vi "ResetBoard.vi"() -> ()   [LabVIEW 2020]
uses:
  _controls/hwEntry_actions.ctl
  AIM664LV.lvlib
panel:
  in  "board":u32
  out "error out":errorcluster
  out "Board Control Out":T1 {"SharedMemFree" format="%x"; "GlobalMemFree" format="%x"; "ExpertMode" items=["FDX_EXPERT_MODE", "FDX_DISA_GHOST"]; "PortGoodLink" items=["FDX_NO_LINK", "FDX_GOOD_LINK"]; "PortSpeed" items=["FDX_100MBIT", "FDX_10MBIT", "FDX_AUTO_100MBIT", "FDX_AUTO_10MBIT"]; "PortConfig" items=["FDX_SINGLE", "FDX_REDUNDANT"]}
  in  "BoardControlIn":T2 {"Control" items=["FDX_READ", "FDX_WRITE"]; "Port1ConfigIn" items=["FDX_SINGLE", "FDX_REDUNDANT"]; "Port2ConfigIn" items=["FDX_SINGLE", "FDX_REDUNDANT"]; "Port3ConfigIn" items=["FDX_SINGLE", "FDX_REDUNDANT"]; "Port4ConfigIn" items=["FDX_SINGLE", "FDX_REDUNDANT"]; "Port1SpeedIn" items=["FDX_100MBIT", "FDX_10MBIT", "FDX_AUTO_100MBIT", "FDX_AUTO_10MBIT"]; "Port2SpeedIn" items=["FDX_100MBIT", "FDX_10MBIT", "FDX_AUTO_100MBIT", "FDX_AUTO_10MBIT"]; "Port3SpeedIn" items=["FDX_100MBIT", "FDX_10MBIT", "FDX_AUTO_100MBIT", "FDX_AUTO_10MBIT"]; "Port4SpeedIn" items=["FDX_100MBIT", "FDX_10MBIT", "FDX_AUTO_100MBIT", "FDX_AUTO_10MBIT"]; "Expert1Mode" items=["FDX_EXPERT_MODE", "FDX_DISA_GHOST"]; "Expert2Mode" items=["FDX_EXPERT_MODE", "FDX_DISA_GHOST"]; "Expert3Mode" items=["FDX_EXPERT_MODE", "FDX_DISA_GHOST"]; "Expert4Mode" items=["FDX_EXPERT_MODE", "FDX_DISA_GHOST"]}
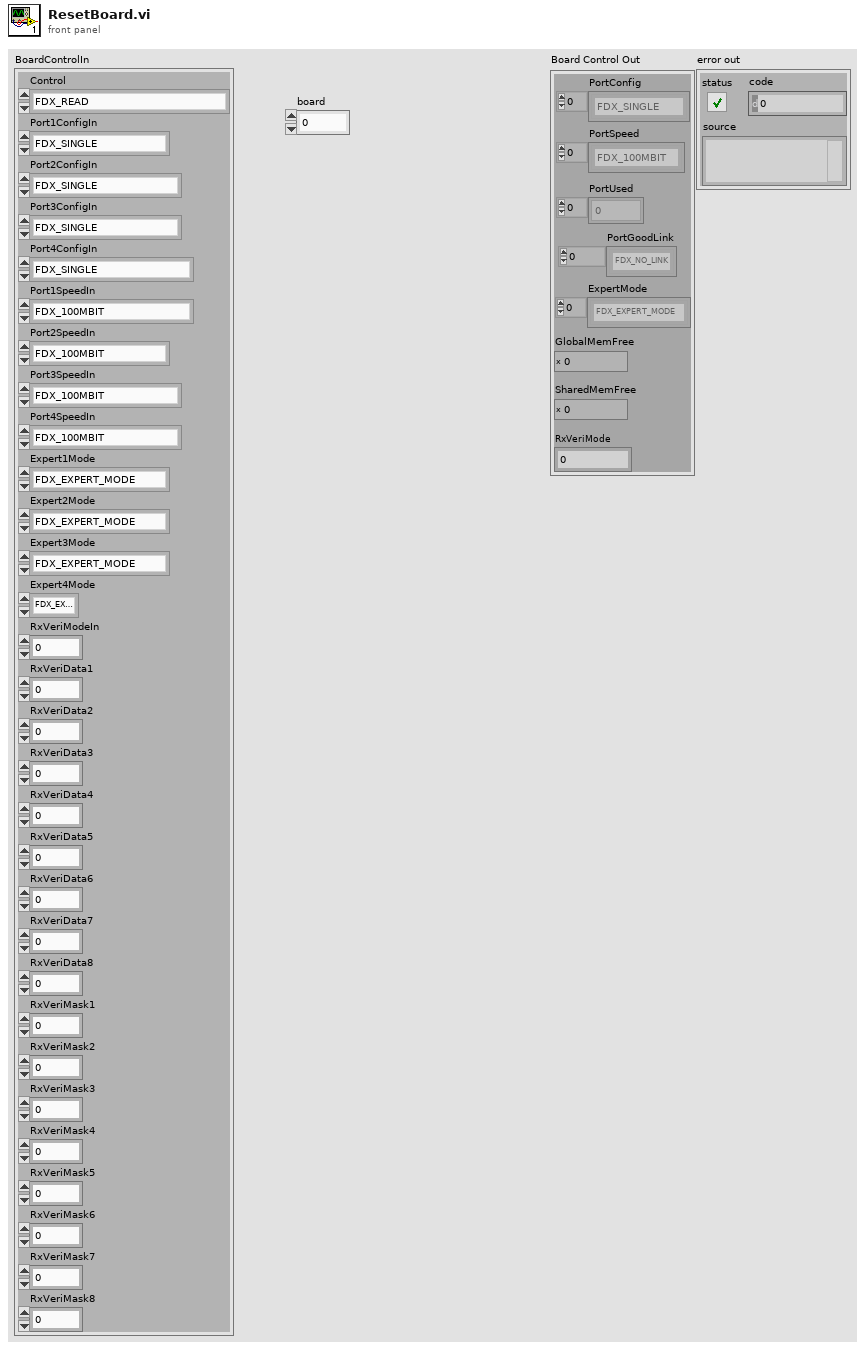
[diagram p1: front panel]
types:
  T1 = cluster{"PortConfig":u32[], "PortSpeed":u32[], "PortUsed":u32[], "PortGoodLink":u32[], "ExpertMode":u32[], "GlobalMemFree":u32, "SharedMemFree":u32, "RxVeriMode":u32}
  T2 = cluster{"Control":u32, "Port1ConfigIn":u32, "Port2ConfigIn":u32, "Port3ConfigIn":u32, "Port4ConfigIn":u32, "Port1SpeedIn":u32, "Port2SpeedIn":u32, "Port3SpeedIn":u32, "Port4SpeedIn":u32, "Expert1Mode":u32, "Expert2Mode":u32, "Expert3Mode":u32, "Expert4Mode":u32, "RxVeriModeIn":u32, "RxVeriData1":u32, "RxVeriData2":u32, "RxVeriData3":u32, "RxVeriData4":u32, "RxVeriData5":u32, "RxVeriData6":u32, "RxVeriData7":u32, "RxVeriData8":u32, "RxVeriMask1":u32, "RxVeriMask2":u32, "RxVeriMask3":u32, "RxVeriMask4":u32, "RxVeriMask5":u32, "RxVeriMask6":u32, "RxVeriMask7":u32, "RxVeriMask8":u32}
  T3 = typedef "AIM664LV.lvlib/hwEntry_actions.ctl" = enum16{"Init Port", "Init Board", "Relase Port", "Release Board"}
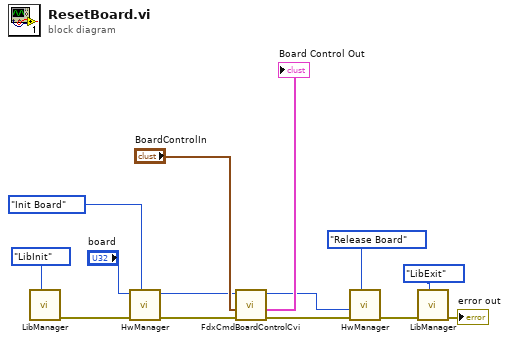
[diagram p0: block diagram]
diagram:
  n1 = call "LibManager.vi"("action"=enum16{"LibInit", "LibExit"}."LibInit") -> ("error out"=w8:errorcluster)  [unwired: 8 in, 2 out]
  n2 = call "HwManager.vi"("action (Init)"=hwEntry_actions."Init Board", "error in (no error)"=w8, "board"="board") -> ("error out"=w7:errorcluster, "InstrumentHandle_board out"=w6:u32)  [unwired: 4 in, 3 out]
  n3 = call "FdxCmdBoardControlCvi.vi"("error in"=w7, "BoardControlIn (read)"="BoardControlIn", "InstrumentHandle_board in"=w6) -> ("error out"=w4:errorcluster, "Board Control Out"=→"Board Control Out":T1, "InstrumentHandle_board out"=w5:u32)  [unwired: 6 in]
  n4 = call "HwManager.vi"("action (Init)"=hwEntry_actions."Release Board", "error in (no error)"=w4, "InstrumentHandle_board in"=w5) -> ("error out"=w11:errorcluster)  [unwired: 4 in, 4 out]
  n5 = call "LibManager.vi"("action"=enum16{"LibInit", "LibExit"}."LibExit", "error in (no error)"=w11) -> ("error out"=→"error out":errorcluster)  [unwired: 7 in, 2 out]
